vi "PCO_SetImageParameters.vi"(7 "dwflags":u32, 8 "error in (no error)":errorcluster {"code" format="%x"}, 9 "wyres":u16, 10 "wxres":u16, 11 "ph":u64) -> (0 "error out":errorcluster {"code" format="%x"}, 2 "ErrorMessage":i32 format="%x", 3 "ph out":u64)   [LabVIEW 2019, in "SDK.lvlib" / "GeneralCameraControl.lvlib"]
doc: "<b>Description:</b>\nThis function does set the image parameters for internal allocated resources. This function must be called, before an image transfer is started from the camera and the image size has been changed since the last PCO_ArmCamera call, this does also include setting a new segment for image readout of the camera internal memory (CamRam). The size parameters are adapted internally, if Meta Data mode or Soft ROI are enabled. In case Soft ROI, see PCO_EnableSoftROI, is in use, dwFlags parameter must be set according to the subsequent program sequence, to ensure that the correct Soft ROI parameters are used. If next images will be transferred from a recording camera, flag IMAGEPARAMETERS_READ_WHILE_RECORDING must be set. If next action is to readout images from the camera internal memory, flag IMAGEPARAMETERS_READ_FROM_SEGMENTS must be set.\n\n<b>Supported camera type:</b>\nAll cameras\n\n<b>Descriptor dependency:</b>\nNone"
uses:
  GeneralCameraControl.lvlib
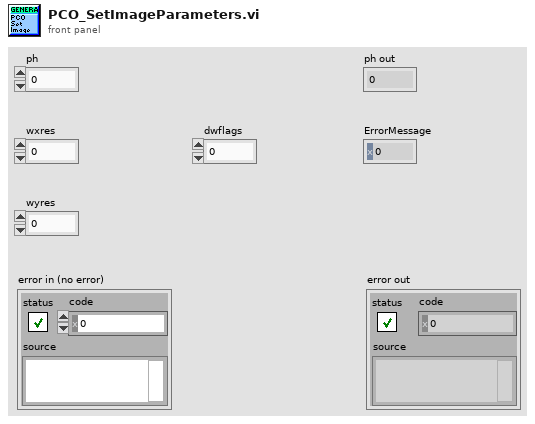
[diagram p1: front panel]
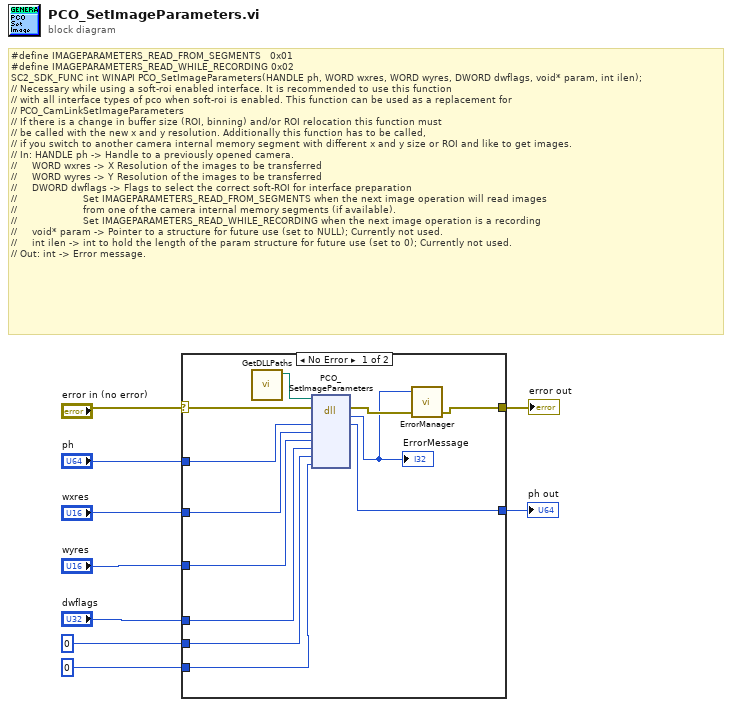
[diagram p0: block diagram]
diagram:
  # "#define IMAGEPARAMETERS_READ_FROM_SEGMENTS   0x01\n#define IMAGEPARAMETERS_READ_WHILE_RECORDING 0x02\nSC2_SDK_FUNC int WINAPI PCO_SetImageParameters(HANDLE ph, WORD wxres, WORD wyres, DWORD dwflags, void* param, int ilen);\n// Necessary while using a soft-roi enabled interface. It is recommended to use this function\n// with all interface types of pco when soft-roi is enabled. This function can be used as a replacement for\n// PCO_CamLinkSetImageParameters\n// If there is a change in buffer size (ROI, binning) and/or ROI relocation this function must\n// be called with the new x and y resolution. Additionally this function has to be called,\n// if you switch to another camera internal memory segment with different x and y size or ROI and like to get images.\n// In: HANDLE ph -> Handle to a previously opened camera.\n//     WORD wxres -> X Resolution of the images to be transferred\n//     WORD wyres -> Y Resolution of the images to be transferred\n//     DWORD dwflags -> Flags to select the correct soft-ROI for interface preparation\n//                      Set IMAGEPARAMETERS_READ_FROM_SEGMENTS when the next image operation will read images\n//                      from one of the camera internal memory segments (if available).\n//                      Set IMAGEPARAMETERS_READ_WHILE_RECORDING when the next image operation is a recording\n//     void* param -> Pointer to a structure for future use (set to NULL); Currently not used.\n//     int ilen -> int to hold the length of the param structure for future use (set to 0); Currently not used.\n// Out: int -> Error message."
  n1 = case shown="No Error" "error in (no error)" {
    selector: "error in (no error)" -> [w17 w23]
    tunnel: "ph" -> [w21 w22]
    tunnel: [w20 w22] -> w8
    tunnel: [w18 w23] -> w7
    tunnel: u64 0 ("param") -> [w15 _]
    tunnel: "dwflags" -> [w14 _]
    tunnel: "wyres" -> [w13 _]
    tunnel: "wxres" -> [w12 _]
    tunnel: 0 ("ilen") -> [w11 _]
    frame No Error {
      n2 = call "GetDLLPaths.vi"() -> ("SC2_Cam_Path"=w10:path)  [unwired: 8 in, 3 out]
      n3 = dll-call lib="?" fn="PCO_SetImageParameters"(path in=w10, error in=w17, "ph"=w21, "wxres"=w12, "wyres"=w13, "dwflags"=w14, "param"=w15, "ilen"=w11) -> (error out=w19:errorcluster, "return type"=w16:i32, "ph"=w20:u64)  [unwired: 6 in, 1 out]
      "ErrorMessage" <- w16
      n4 = call "ErrorManager.vi"("error in (no error)"=w19, "error code"=w16) -> ("error out"=w18:errorcluster)  [unwired: 2 in, 1 out]
    }
    frame Error {
    }
  }
  "ph out" <- w8
  "error out" <- w7
